vi "fetch_and_translate_triggers.vi"(8 "error in (no error)":errorcluster, 11 "InstrumentDL090324 in":refnum<class "InstrumentDL090324.lvclass">) -> (0 "error out":errorcluster, 1 "sender TLC type":T1, 2 "statechart trigger":T2, 3 "InstrumentDL090324 out":refnum<class "InstrumentDL090324.lvclass">)   [LabVIEW 2010, in "InstrumentDL090324.lvclass"]
uses:
  InstrumentDL090324.lvclass
  internal_trigger_enum.ctl
  common/enumerations/top-level_component_type_enum.ctl
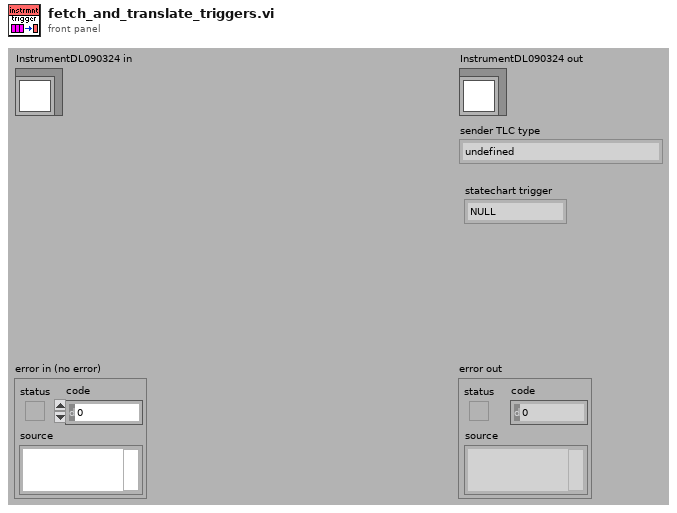
[diagram p1: front panel]
types:
  T1 = typedef "top-level_component_type_enum.ctl" = enum16{"undefined", "ImagingMode", "ScanHead", "DAQ", "ImageAssembler", "Display", "DataCollection", "Analyser", "Stimulator", "ExperimentController", "Instrument", "Stage"}
  T2 = typedef "InstrumentDL090324.lvclass/internal_trigger_enum.ctl" = enum16{"NULL", "initialise", "terminate", "start", "stop"}
  T3 = typedef "GenericToplevelComponent.lvclass/common_trigger_enum.ctl" = enum16{"NULL", "initialise", "terminate", "fetch command", "fetch data", "attach observer", "register as observer", "detach observer", "acknowledge", "start", "stop", "sweep started", "sweep finished", "experiment started", "experiment stopped"}
  T4 = typedef "trigger_type_enum.ctl" = enum8{"external", "internal", "common"}
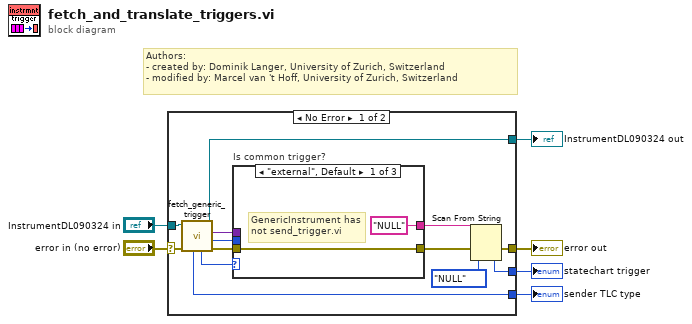
[diagram p0: block diagram]
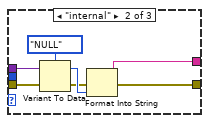
[diagram p2: hidden frame]
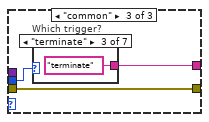
[diagram p3: hidden frame]
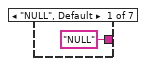
[diagram p4: hidden frame]
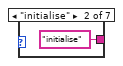
[diagram p5: hidden frame]
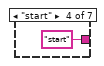
[diagram p6: hidden frame]
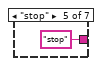
[diagram p7: hidden frame]
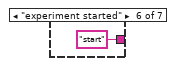
[diagram p8: hidden frame]
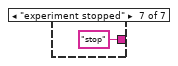
[diagram p9: hidden frame]
diagram:
  # "Authors: \n- created by: Dominik Langer, University of Zurich, Switzerland\n- modified by: Marcel van 't Hoff, University of Zurich, Switzerland"
  n1 = case shown="No Error" "error in (no error)" {
    selector: "error in (no error)" -> [w19 w40]
    tunnel: [w10 w40] -> w5
    tunnel: [w13 w39] -> w3
    tunnel: "InstrumentDL090324 in" -> [w14 w39]
    tunnel: [w8 _] -> w2
    tunnel: [w12 _] -> w1
    frame No Error {
      n2 = call-dynamic "fetch_generic_trigger.vi"("error in (no error)"=w19, "GenericToplevelComponent in"=w14) -> ("error out"=w17:errorcluster, "common trigger"=w15:T3, "trigger"=w18:variant, "GenericToplevelComponent out"=w13:refnum<class "InstrumentDL090324.lvclass">, "trigger type"=w16:T4, "sender TLC type"=w12:T1)  [unwired: 3 in, 1 out]
      n3 = case "Is common trigger?" shown="\"external\", Default" w16 {
        tunnel: w18 -> [_ w27 _]
        tunnel: w17 -> [w21 w26 w31]
        tunnel: [w21 w22 w31] -> w9
        tunnel: w15 -> [_ _ w30]
        tunnel: ["NULL" w24 w29] -> w7
        frame "external", Default {
          # "GenericInstrument has not send_trigger.vi"
        }
        frame "internal" {
          n4 = Variant To Data(error in=w26, Variant=w27, type=internal_trigger_enum."NULL" ("last trigger")) -> (error out=w23:errorcluster, data=w25:T2)
          n5 = Format Into String(error in=w23, w25) -> (resulting string=w24:string, error out=w22:errorcluster)  [unwired: 2 in]
        }
        frame "common" {
          n6 = case "Which trigger?" shown="\"terminate\"" w30 {
            tunnel: ["NULL" "initialise" "terminate" "start" "stop" "start" "stop"] -> w29
            frame "NULL", Default {
            }
            frame "initialise" {
            }
            frame "terminate" {
            }
            frame "start" {
            }
            frame "stop" {
            }
            frame "experiment started" {
            }
            frame "experiment stopped" {
            }
          }
        }
      }
      n7 = Scan From String(input string=w7, error in=w9, default 1=internal_trigger_enum."NULL" ("statechart trigger")) -> (error out=w10:errorcluster, output 1=w8:T2)  [unwired: 2 in, 2 out]
    }
    frame Error {
    }
  }
  "error out" <- w5
  "InstrumentDL090324 out" <- w3
  "statechart trigger" <- w2
  "sender TLC type" <- w1
